vi "GammaGovernorHost.vi"() -> ()   [LabVIEW 2014]
uses:
  <vilib>/userdefined/High Color/nirio_resource_hc.ctl
  <vilib>/Analysis/2dsp.llb/Decimate (single shot, DBL).vi
  <vilib>/Analysis/baseanly.llb/Vector x A.vi
  <vilib>/FPGAPlugInAG/USB-7845R/niLvFpga_Open_USB-7845R.vi
  <vilib>/rvi/interface/common/dynamic/niFpgaDynamicAddResources.vi
  <vilib>/FPGAPlugInAG/Dynamic/niLvFpga_Download_Dynamic.vi
  <vilib>/FPGAPlugInAG/Dynamic/niLvFpga_Run_Dynamic.vi
  <vilib>/Utility/error.llb/Error Cluster From Error Code.vi
  <vilib>/rvi/errors/niLvFpgaAdjustHostInterfaceError.vi
  <vilib>/Analysis/3filter.llb/Butterworth Filter (DBL).vi
  <vilib>/express/express analysis/Spectral/Block/exnSpectralBlock spectral measurements PSD poly.vi
  <vilib>/express/express analysis/Spectral/Block/exnSpectralBlock spectral measurements PSD WFM.vi
  <vilib>/FPGAPlugInAG/Dynamic/niLvFpga_Close_Dynamic.vi
  <vilib>/rvi/interface/nirviOpenFPGA/nirviOpenFPGA.xnode
  C:/Users/Public/Documents/National Instruments/DBH_VIs/CLCommander/FPGA Bitfiles/GammaGovernor_FPGATarget_ClosedLoopComman_V1+uTFggb4c.lvbitx
  C:/Users/Public/Documents/National Instruments/DBH_VIs/CLCommander/GammaGovernorTarget.vi
  <vilib>/rvi/interface/nirviMethod/nirviMethod.xnode
  <vilib>/express/express analysis/Spectral/XNode/ExpressSpectralMeasurementsBlockNode.xnode
  <vilib>/rvi/interface/nirviCloseFPGA/nirviCloseFPGA.xnode
  <vilib>/Analysis/NI_AALPro.lvlib
  <vilib>/Analysis/NI_AALBase.lvlib
  <vilib>/FPGAPlugInAG/Dynamic/niLvFpga_ReadFifo_Dynamic.vi
  <vilib>/rvi/errors/niLvFpgaMergeErrorWithErrorCode.vi
panel:
  in  "Stop Gamma Governor":bool
  in  "FPGA Target Device":T1
  out "Filtered Trigger Average Left":cluster{waveform(dbl), waveform(dbl)}(graph)
  in  "high cutoff freq: fh":dbl=100.0 format="%#_13g"
  in  "low cutoff freq: fl":dbl=30.0 format="%#_13g"
  out "Filtered Trigger Average Right":cluster{waveform(dbl), waveform(dbl)}(graph)
  in  "Store":bool
  in  "Reset":bool
  out "Spectrogram Left":dbl[][](graph)
  out "Spectrogram Right":dbl[][](graph)
  out "Monitoring signals":T2(graph)
  out "size(s)":i32
  out "Numeric":i32
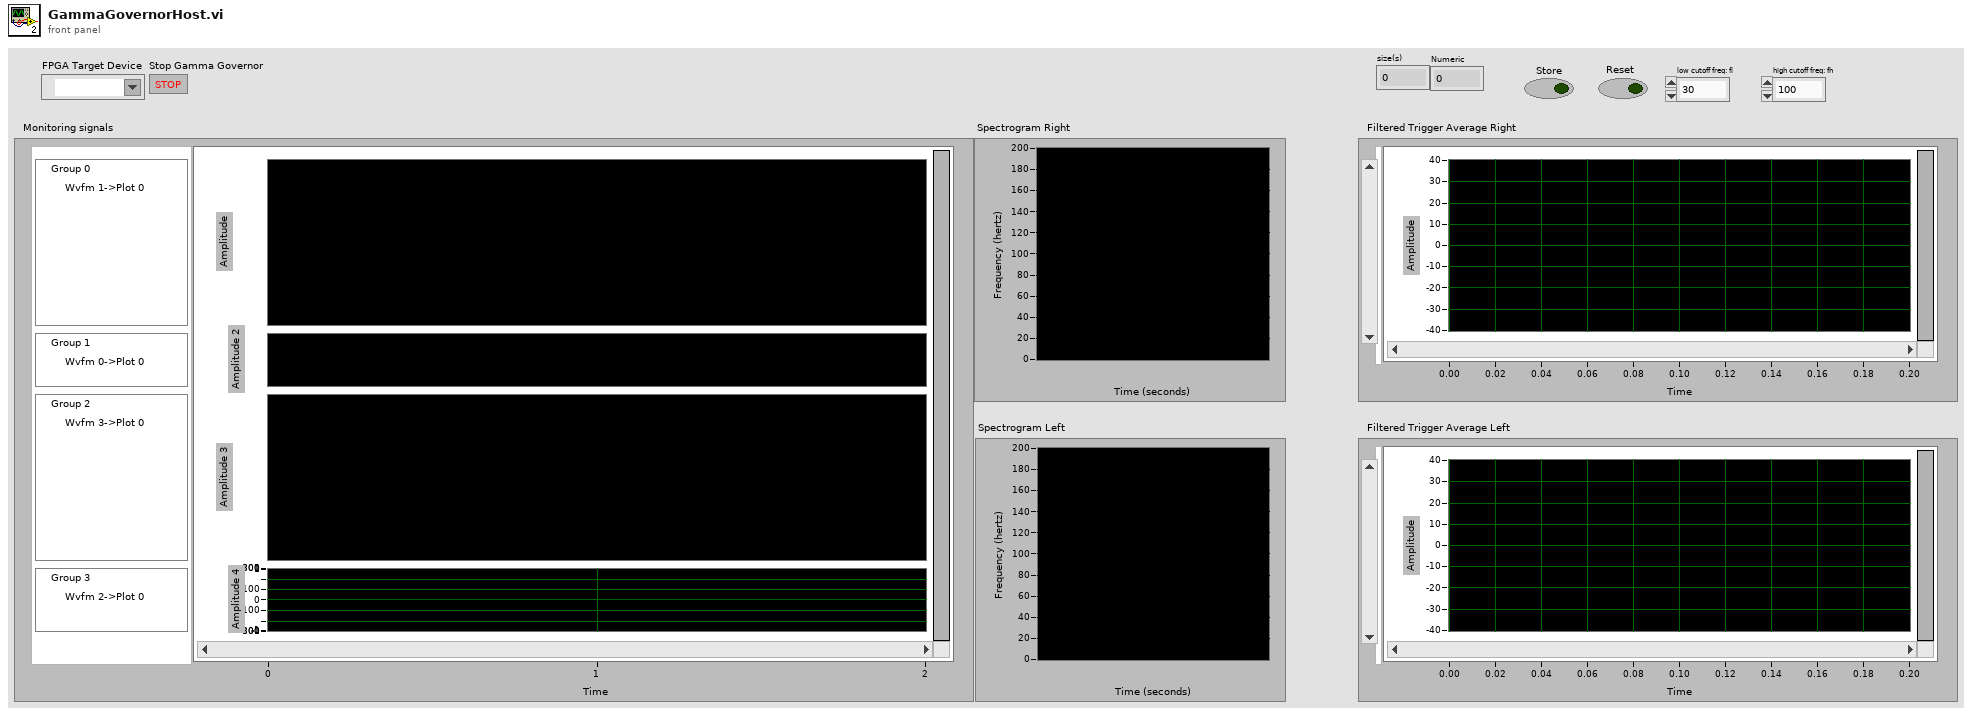
[diagram p1: front panel]
types:
  T1 = typedef "nirio_resource_hc.ctl" = tag
  T2 = cluster{waveform(u8), waveform(dbl), waveform(u8), waveform(dbl)}
  T3 = cluster{"averaging mode":u16, "weighting mode":u16, "number of averages":u32}
  T4 = cluster{"dB On (F)":bool, "unwrap phase (F)":bool, "convert to degree (F)":bool}
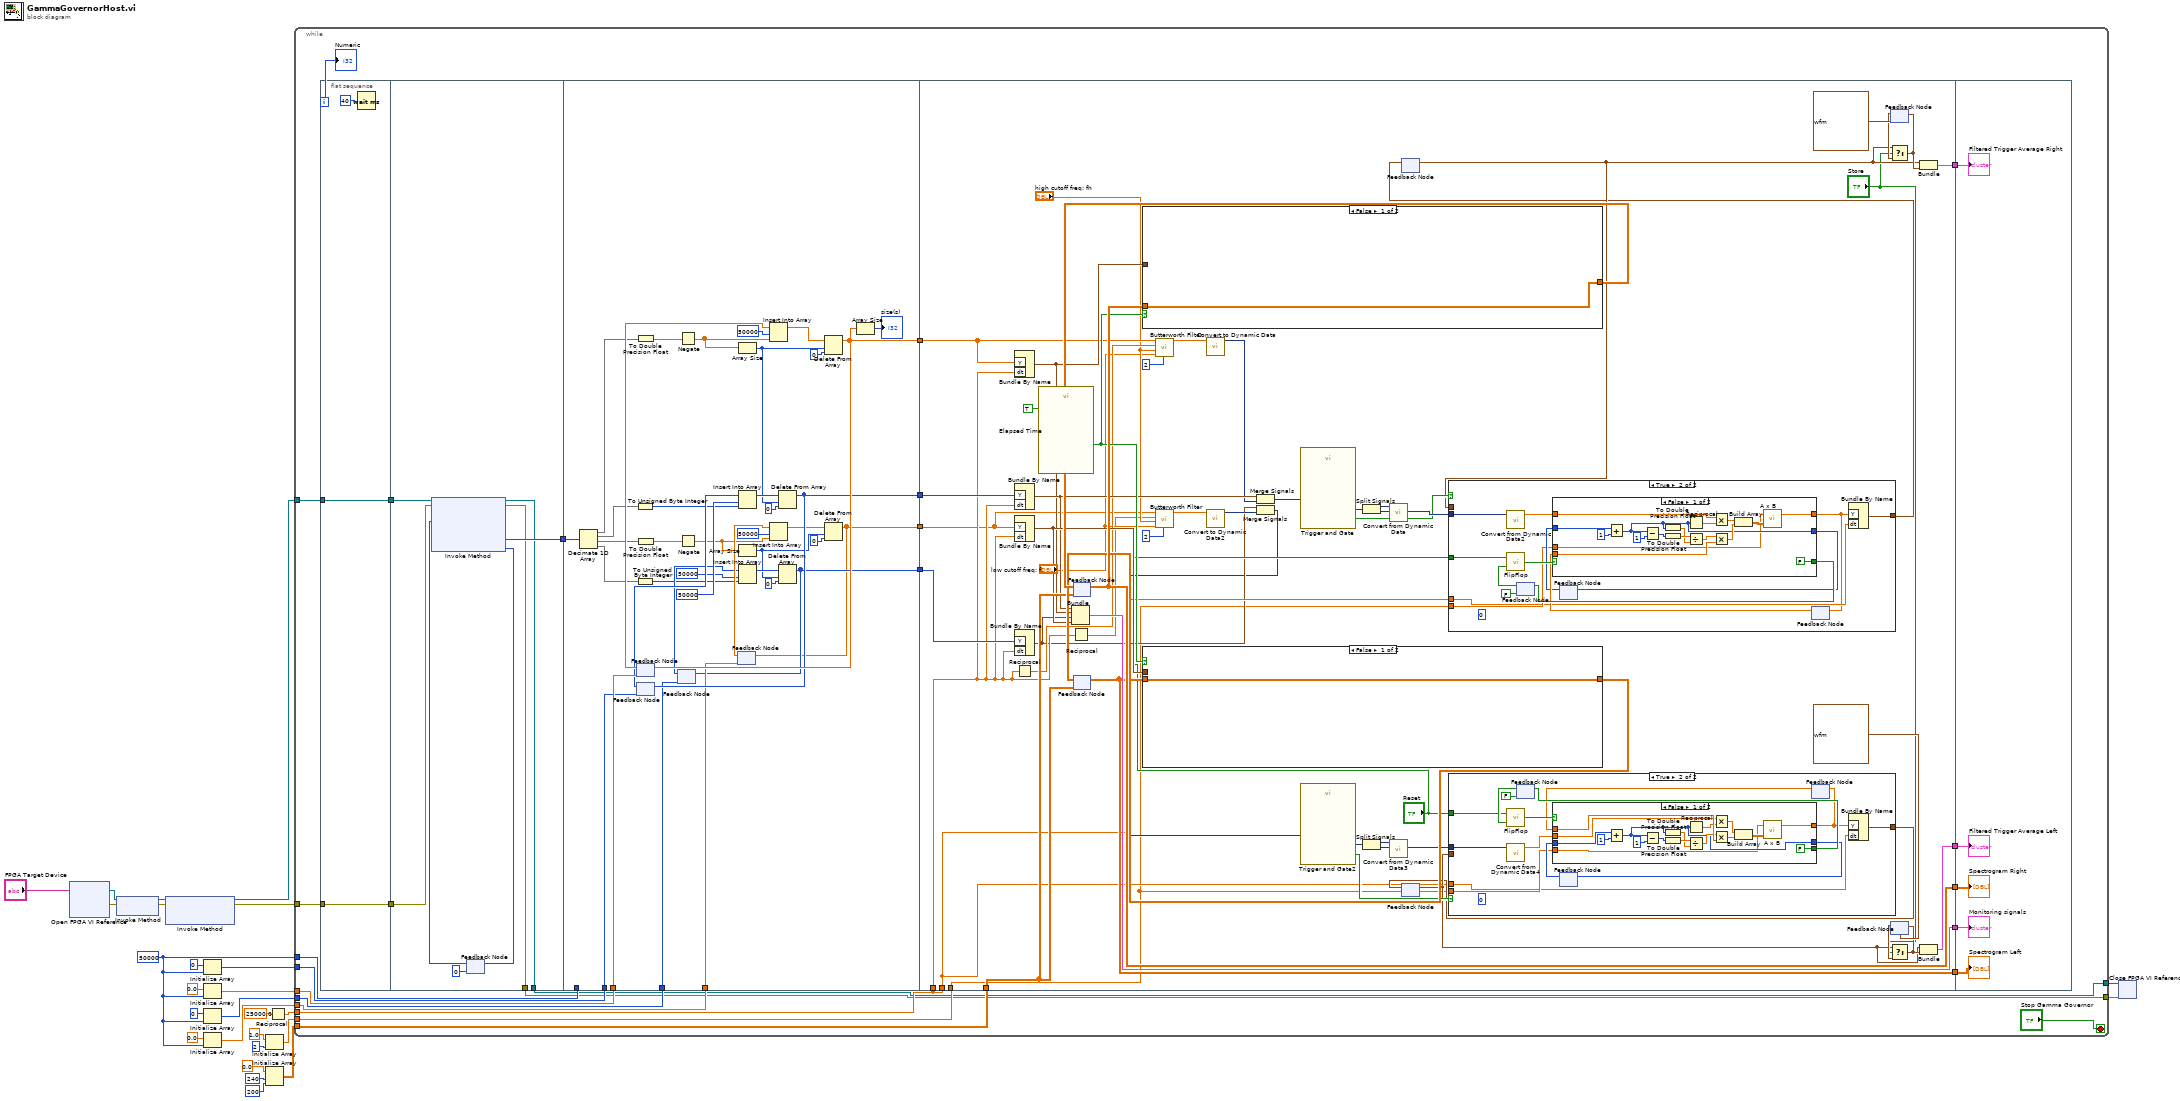
[diagram p0: block diagram]
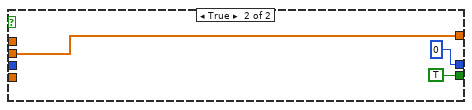
[diagram p3: hidden frame]
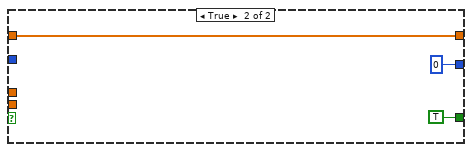
[diagram p5: hidden frame]
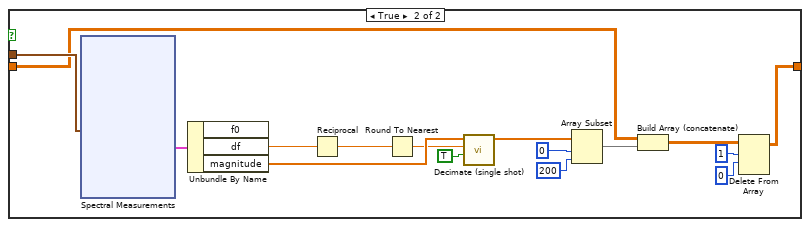
[diagram p6: hidden frame]
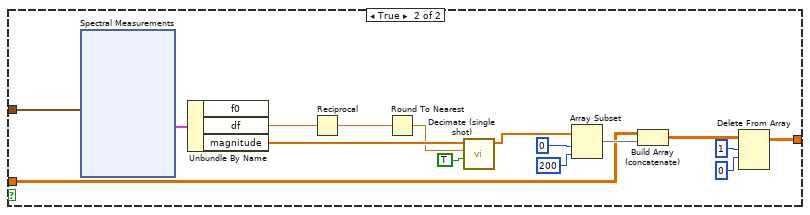
[diagram p7: hidden frame]
diagram:
  w15 = 50000 ("dimension size")
  n1 = xnode "Open FPGA VI Reference"("resource name"="FPGA Target Device") -> ("FPGA VI Reference Out"=w6:refnum<k20>, "error out"=w5:errorcluster)  [unwired: 1 in]
  n2 = xnode "Invoke Method"("FPGA VI Reference In"=w6, "error in"=w5) -> ("FPGA VI Reference Out"=w4:refnum<k20>, "error out"=w3:errorcluster)
  n3 = xnode "Invoke Method"("FPGA VI Reference In"=w4, "error in"=w3) -> ("FPGA VI Reference Out"=w26:refnum<k20>, "error out"=w27:errorcluster)  [unwired: 1 in]
  n4 = Initialize Array(u8 0 ("element"), w15) -> (w20:u8[])
  n5 = Initialize Array(0.0 ("element"), w15) -> (w24:dbl[])
  n6 = Initialize Array(u8 0 ("element"), w15) -> (w17:u8[])
  n7 = Initialize Array(0.0 ("element"), w15) -> (w16:dbl[])
  n8 = Initialize Array(1.0 ("element"), 2 ("dimension size")) -> (w8:dbl[])
  n9 = Initialize Array(0.0 ("element"), 240 ("dimension size"), 200 ("dimension size")) -> (w11:dbl[][])
  n10 = Reciprocal(x=25000.0) -> (1/x=w22:dbl)
  n11 = while {
    tunnel: w27 -> [w51]
    tunnel: w26 -> [w52]
    tunnel: w24 -> [w49]
    tunnel: w15 -> [w48]
    tunnel: w22 -> [w33]
    tunnel: w20 -> [w46]
    tunnel: w17 -> [w41]
    tunnel: w16 -> [w40]
    tunnel: w11 -> [w37]
    tunnel: w8 -> [w34]
    tunnel: [w29] -> w2
    tunnel: [w28] -> w1
    i -> [w53]
    stop <- "Stop Gamma Governor" stop-if-true
    n12 = flat-sequence {
      tunnel: w52 -> [w56]
      tunnel: w51 -> [w55]
      tunnel: [w56] -> w43
      tunnel: [w55] -> w42
      tunnel: [w64] -> w50
      tunnel: w43 -> [w63]
      tunnel: w42 -> [w62]
      tunnel: [w58] -> w29
      tunnel: [w57] -> w28
      tunnel: w50 -> [w102]
      tunnel: w49 -> [w101]
      tunnel: w48 -> [_]
      tunnel: [w96] -> w47
      tunnel: w46 -> [w90]
      tunnel: [w87] -> w45
      tunnel: w41 -> [w68]
      tunnel: w40 -> [w67]
      tunnel: [w66] -> w39
      tunnel: [w65] -> w38
      tunnel: w33 -> [w111]
      tunnel: w47 -> [w129]
      tunnel: w45 -> [w155]
      tunnel: [w154] -> w44
      tunnel: w39 -> [w153]
      tunnel: w38 -> [w109]
      tunnel: w37 -> [w148]
      tunnel: [w150] -> w36
      tunnel: [w145] -> w35
      tunnel: w34 -> [w104]
      tunnel: w33 -> [w117]
      tunnel: [w132] -> w32
      tunnel: [w103] -> w31
      tunnel: w44 -> [w284]
      tunnel: w36 -> [w283]
      tunnel: w35 -> [w282]
      tunnel: w32 -> [w281]
      tunnel: w31 -> [w280]
      frame #0 {
        n13 = Wait (ms)(milliseconds to wait=u32 40) -> ()  [unwired: 1 out]
      }
      frame #1 {
        n14 = feedback #1(u32 0 ("Elements Remaining")) -> (w60:u32)
        n15 = xnode "Invoke Method"("FPGA VI Reference In"=w63, "error in"=w62, "Number of Elements"=w60) -> ("FPGA VI Reference Out"=w58:refnum<k20>, "error out"=w57:errorcluster, "Data"=w64:i16[], "Elements Remaining"=w61:u32)  [unwired: 1 in]
        n16 = feedback-in #1(w61) -> ()
      }
      frame #2 {
        n17 = Decimate 1D Array(w102) -> (w84:i16[], w83:i16[], w70:i16[], w69:i16[])
        n18 = To Unsigned Byte Integer(number=w83) -> (unsigned 8bit integer=w88:u8[])
        n19 = To Unsigned Byte Integer(number=w69) -> (unsigned 8bit integer=w73:u8[])
        n20 = To Double Precision Float(number=w84) -> (double precision float=w86:dbl[])
        n21 = To Double Precision Float(number=w70) -> (double precision float=w72:dbl[])
        n22 = feedback #2(w101) -> (w100:dbl[])
        n23 = feedback #3(w90) -> (w94:u8[])
        n24 = feedback #4(w68) -> (w78:u8[])
        n25 = Negate(x=w86) -> (-x=w85:dbl[])
        n26 = Negate(x=w72) -> (-x=w71:dbl[])
        n27 = feedback #5(w67) -> (w82:dbl[])
        n28 = Array Size(array=w85) -> (size(s)=w89:i32)
        n29 = Insert Into Array(array=w94, index=50000, new element=w88) -> (w91:u8[])
        n30 = Array Size(array=w71) -> (size(s)=w74:i32)
        n31 = Insert Into Array(array=w78, index=50000, new element=w73) -> (w75:u8[])
        n32 = Insert Into Array(array=w100, index=50000, new element=w85) -> (w97:dbl[])
        n33 = Insert Into Array(array=w82, index=50000, new element=w71) -> (w79:dbl[])
        n34 = Delete From Array(array=w91, length=w89, index=0) -> (array with subset deleted=w87:u8[])  [unwired: 1 out]
        n35 = feedback-in #3(w87) -> ()
        n36 = Delete From Array(array=w75, length=w74, index=0) -> (array with subset deleted=w66:u8[])  [unwired: 1 out]
        n37 = feedback-in #4(w66) -> ()
        n38 = Delete From Array(array=w97, length=w89, index=0) -> (array with subset deleted=w96:dbl[])  [unwired: 1 out]
        n39 = feedback-in #2(w96) -> ()
        n40 = Delete From Array(array=w79, length=w74, index=0) -> (array with subset deleted=w65:dbl[])  [unwired: 1 out]
        n41 = feedback-in #5(w65) -> ()
        n42 = Array Size(array=w96) -> (size(s)=→"size(s)":i32)
      }
      frame #3 {
        n43 = Bundle By Name("Y"=w129, "dt"=w111) -> (w142:waveform(dbl))  [unwired: 1 in]
        n44 = Bundle By Name("Y"=w155, "dt"=w111) -> (w143:waveform(u8))  [unwired: 1 in]
        n45 = Bundle By Name("Y"=w109, "dt"=w111) -> (w147:waveform(dbl))  [unwired: 1 in]
        n46 = Bundle By Name("Y"=w153, "dt"=w111) -> (w106:waveform(u8))  [unwired: 1 in]
        n47 = Reciprocal(x=w111) -> (1/x=w131:dbl)
        n48 = call "Elapsed Time"("Auto Reset"=TRUE) -> ("Time has Elapsed"=w146:bool)  [unwired: 11 in, 7 out]
        n49 = Bundle(w143, w142, w106, w147) -> (w154:T2)  [unwired: 1 in]
        n50 = Reciprocal(x=w111) -> (1/x=w110:dbl)
        n51 = feedback #6(w148) -> (w150:dbl[][])
        n52 = feedback #7(w148) -> (w145:dbl[][])
        n53 = case shown="False" w146 {
          tunnel: w142 -> [_ w260]
          tunnel: [w253 w255] -> w151
          tunnel: w150 -> [w253 w254]
          frame False {
          }
          frame True {
            n54 = xnode "Spectral Measurements"("Signals"=w260) -> ("PSD"=w261:cluster{"f0":dbl, "df":dbl, "magnitude":dbl[]})  [unwired: 2 in, 2 out]
            n55 = Unbundle By Name(w261) -> ("df"=w262:dbl, "magnitude"=w266:dbl[])  [unwired: 1 out]
            n56 = Reciprocal(x=w262) -> (1/x=w263:dbl)
            n57 = Round To Nearest(number=w263) -> (nearest integer value=w264:dbl)
            n58 = call-poly <vilib>:"Decimate (single shot).vi"("averaging"=TRUE, "decimating factor"=w264, "X"=w266) -> ("Decimated Array"=w267:dbl[])  [unwired: 7 in, 1 out]
            n59 = Array Subset(array=w267, index=0, length=200) -> (w259:dbl[])
            n60 = Build Array (concatenate)(w254, w259) -> (w258:dbl[][])
            n61 = Delete From Array(array=w258, length=1, index (row)=0) -> (array with subset deleted=w255:dbl[][])  [unwired: 1 in, 1 out]
          }
        }
        n62 = feedback-in #6(w151) -> ()
        n63 = case shown="False" w146 {
          tunnel: [w226 w229] -> w149
          tunnel: w147 -> [_ w228]
          tunnel: w145 -> [w226 w227]
          frame False {
          }
          frame True {
            n64 = xnode "Spectral Measurements"("Signals"=w228) -> ("PSD"=w234:cluster{"f0":dbl, "df":dbl, "magnitude":dbl[]})  [unwired: 2 in, 2 out]
            n65 = Unbundle By Name(w234) -> ("df"=w235:dbl, "magnitude"=w239:dbl[])  [unwired: 1 out]
            n66 = Reciprocal(x=w235) -> (1/x=w236:dbl)
            n67 = Round To Nearest(number=w236) -> (nearest integer value=w237:dbl)
            n68 = call-poly <vilib>:"Decimate (single shot).vi"("averaging"=TRUE, "decimating factor"=w237, "X"=w239) -> ("Decimated Array"=w240:dbl[])  [unwired: 7 in, 1 out]
            n69 = Array Subset(array=w240, index=0, length=200) -> (w233:dbl[])
            n70 = Build Array (concatenate)(w227, w233) -> (w232:dbl[][])
            n71 = Delete From Array(array=w232, length=1, index (row)=0) -> (array with subset deleted=w229:dbl[][])  [unwired: 1 in, 1 out]
          }
        }
        n72 = feedback-in #7(w149) -> ()
        n73 = call-poly <vilib>:"Butterworth Filter.vi"("order"=2, "low cutoff freq: fl"="low cutoff freq: fl", "high cutoff freq: fh"="high cutoff freq: fh", "sampling freq: fs"=w131, "X"=w129) -> ("Filtered X"=w128:dbl[])  [unwired: 3 in, 1 out]
        n74 = call-poly <vilib>:"Butterworth Filter.vi"("order"=2, "low cutoff freq: fl"="low cutoff freq: fl", "high cutoff freq: fh"="high cutoff freq: fh", "sampling freq: fs"=w110, "X"=w109) -> ("Filtered X"=w107:dbl[])  [unwired: 3 in, 1 out]
        n75 = call "Convert to Dynamic Data"("Array"=w128) -> ("Dynamic Data Type"=w127:dynamicdata)  [unwired: 3 in]
        n76 = call "Convert to Dynamic Data2"("Array"=w107) -> ("Dynamic Data Type"=w108:dynamicdata)  [unwired: 3 in]
        n77 = Merge Signals(w143, w127) -> (w144:dynamicdata)
        n78 = Merge Signals(w106, w108) -> (w105:dynamicdata)
        n79 = call "Trigger and Gate"("Signals"=w144) -> ("Triggered Signals"=w140:dynamicdata, "Data Available"=w138:bool)  [unwired: 7 in, 2 out]
        n80 = call "Trigger and Gate2"("Signals"=w105) -> ("Triggered Signals"=w125:dynamicdata, "Data Available"=w123:bool)  [unwired: 7 in, 2 out]
        n81 = Split Signals(w140) -> (w139:dynamicdata, w141:dynamicdata)  [unwired: 2 in]
        n82 = Split Signals(w125) -> (w124:dynamicdata, w126:dynamicdata)  [unwired: 2 in]
        n83 = call "Convert from Dynamic Data"("Dynamic Data Type"=w139) -> ()  [unwired: 3 in, 1 out]
        n84 = call "Convert from Dynamic Data3"("Dynamic Data Type"=w124) -> ()  [unwired: 3 in, 1 out]
        n85 = feedback #8() -> (w134:waveform(dbl))  [unwired: 1 in]
        n86 = feedback #9() -> (w119:waveform(dbl))  [unwired: 1 in]
        n87 = case shown="True" w138 {
          tunnel: w141 -> [_ w205]
          tunnel: "Reset" -> [_ w198]
          tunnel: w104 -> [_ w196]
          tunnel: w134 -> [w191 _]
          tunnel: [w191 w194] -> w133
          tunnel: w117 -> [_ w193]
          frame False {
          }
          frame True {
            (unwired) 0
            n88 = call "Convert from Dynamic Data2"("Dynamic Data Type"=w205) -> ("Array"=w197:dbl[])  [unwired: 3 in]
            n89 = feedback #10(FALSE) -> (w202:bool)
            n90 = call "FlipFlop.vi"("Reset"=w202, "Set"=w198) -> ("Ouput"=w204:bool)
            n91 = feedback #11() -> (w199:i32)  [unwired: 1 in]
            n92 = feedback #12() -> (w200:dbl[])  [unwired: 1 in]
            n93 = case shown="False" w204 {
              tunnel: [FALSE TRUE] -> w203
              tunnel: w197 -> [w212 w224]
              tunnel: [w206 w224] -> w192
              tunnel: w200 -> [w219 _]
              tunnel: [w210 0] -> w195
              tunnel: w199 -> [w220 _]
              tunnel: w196 -> [w207 _]
              frame False {
                n94 = Add(x=w220, y=1) -> (x+y=w210:i32)
                n95 = Subtract(x=w210, y=1) -> (x-y=w217:i32)
                n96 = To Double Precision Float(number=w210) -> (double precision float=w215:dbl)
                n97 = To Double Precision Float(number=w217) -> (double precision float=w216:dbl)
                n98 = Reciprocal(x=w210) -> (1/x=w211:dbl)
                n99 = Divide(x=w216, y=w215) -> (x/y=w214:dbl)
                n100 = Multiply(x=w212, y=w211) -> (x*y=w209:dbl[])
                n101 = Multiply ("Multiply.vi")(x=w214, y=w219) -> (x*y=w213:dbl[])
                n102 = Build Array(w209, w213) -> (w208:dbl[][])
                n103 = call-poly <vilib>:"A x B.vi"("Matrix A"=w208, "Vector V'"=w207) -> ("V' x A"=w206:dbl[])  [unwired: 1 out]
              }
              frame True {
              }
            }
            n104 = feedback-in #10(w203) -> ()
            n105 = feedback-in #11(w195) -> ()
            n106 = feedback-in #12(w192) -> ()
            n107 = Bundle By Name("Y"=w192, "dt"=w193) -> (w194:waveform(dbl))  [unwired: 1 in]
          }
        }
        n108 = feedback-in #8(w133) -> ()
        n109 = case shown="True" w123 {
          tunnel: w126 -> [_ w170]
          tunnel: "Reset" -> [_ w163]
          tunnel: w104 -> [_ w161]
          tunnel: w119 -> [w156 _]
          tunnel: [w156 w159] -> w118
          tunnel: w117 -> [_ w158]
          frame False {
          }
          frame True {
            (unwired) 0
            n110 = call "Convert from Dynamic Data4"("Dynamic Data Type"=w170) -> ("Array"=w162:dbl[])  [unwired: 3 in]
            n111 = feedback #13(FALSE) -> (w167:bool)
            n112 = call "FlipFlop.vi"("Reset"=w167, "Set"=w163) -> ("Ouput"=w169:bool)
            n113 = feedback #14() -> (w164:i32)  [unwired: 1 in]
            n114 = feedback #15() -> (w165:dbl[])  [unwired: 1 in]
            n115 = case shown="False" w169 {
              tunnel: [FALSE TRUE] -> w168
              tunnel: w162 -> [w177 w189]
              tunnel: [w171 w189] -> w157
              tunnel: w165 -> [w184 _]
              tunnel: [w175 0] -> w160
              tunnel: w164 -> [w185 _]
              tunnel: w161 -> [w172 _]
              frame False {
                n116 = Add(x=w185, y=1) -> (x+y=w175:i32)
                n117 = Subtract(x=w175, y=1) -> (x-y=w182:i32)
                n118 = To Double Precision Float(number=w175) -> (double precision float=w180:dbl)
                n119 = To Double Precision Float(number=w182) -> (double precision float=w181:dbl)
                n120 = Reciprocal(x=w175) -> (1/x=w176:dbl)
                n121 = Divide(x=w181, y=w180) -> (x/y=w179:dbl)
                n122 = Multiply(x=w177, y=w176) -> (x*y=w174:dbl[])
                n123 = Multiply ("Multiply.vi")(x=w179, y=w184) -> (x*y=w178:dbl[])
                n124 = Build Array(w174, w178) -> (w173:dbl[][])
                n125 = call-poly <vilib>:"A x B.vi"("Matrix A"=w173, "Vector V'"=w172) -> ("V' x A"=w171:dbl[])  [unwired: 1 out]
              }
              frame True {
              }
            }
            n126 = feedback-in #13(w168) -> ()
            n127 = feedback-in #14(w160) -> ()
            n128 = feedback-in #15(w157) -> ()
            n129 = Bundle By Name("Y"=w157, "dt"=w158) -> (w159:waveform(dbl))  [unwired: 1 in]
          }
        }
        n130 = feedback-in #9(w118) -> ()
        n131 = feedback #16(waveform(dbl) {"t0"=timestamp(0 s since 1904-01-01), "dt"=1.0, "Y"=[]}) -> (w136:waveform(dbl))
        n132 = Select(t=w134, s="Store", f=w136) -> (s? t:f=w135:waveform(dbl))
        n133 = feedback-in #16(w135) -> ()
        n134 = feedback #17(waveform(dbl) {"t0"=timestamp(0 s since 1904-01-01), "dt"=1.0, "Y"=[]}) -> (w121:waveform(dbl))
        n135 = Select(t=w119, s="Store", f=w121) -> (s? t:f=w120:waveform(dbl))
        n136 = feedback-in #17(w120) -> ()
        n137 = Bundle(w134, w135) -> (w132:cluster{waveform(dbl), waveform(dbl)})  [unwired: 1 in]
        n138 = Bundle(w119, w120) -> (w103:cluster{waveform(dbl), waveform(dbl)})  [unwired: 1 in]
      }
      frame #4 {
        "Monitoring signals" <- w284
        "Spectrogram Right" <- w283
        "Spectrogram Left" <- w282
        "Filtered Trigger Average Right" <- w281
        "Filtered Trigger Average Left" <- w280
      }
    }
    "Numeric" <- w53
  }
  n139 = xnode "Close FPGA VI Reference"("FPGA VI Reference In"=w2, "error in"=w1) -> ()  [unwired: 1 out]
